vi "PeakAll.vi"(11 "POTTypedCircularBuffer in":refnum<class "ErrorLogBuffer.lvclass">) -> (2 "Copied Buffer":T1[](array[typedef]), 3 "POTTypedCircularBuffer out":refnum<class "ErrorLogBuffer.lvclass">)   [LabVIEW 2024, in "ErrorLogBuffer.lvclass"]
uses:
  ErrorLogBuffer.lvclass
  Type.ctl
  RQMHCore/ErrorReporting/Record/LogRecord.lvclass
  ErrorLogBuffer.lvclass/ErrorLogBuffer.ctl
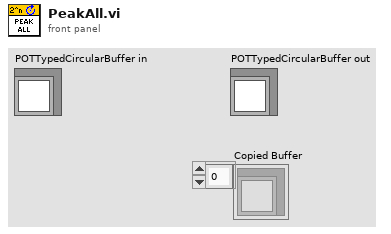
[diagram p1: front panel]
types:
  T1 = typedef "ErrorLogBuffer.lvclass/Type.ctl" = refnum<class "LogRecord.lvclass">
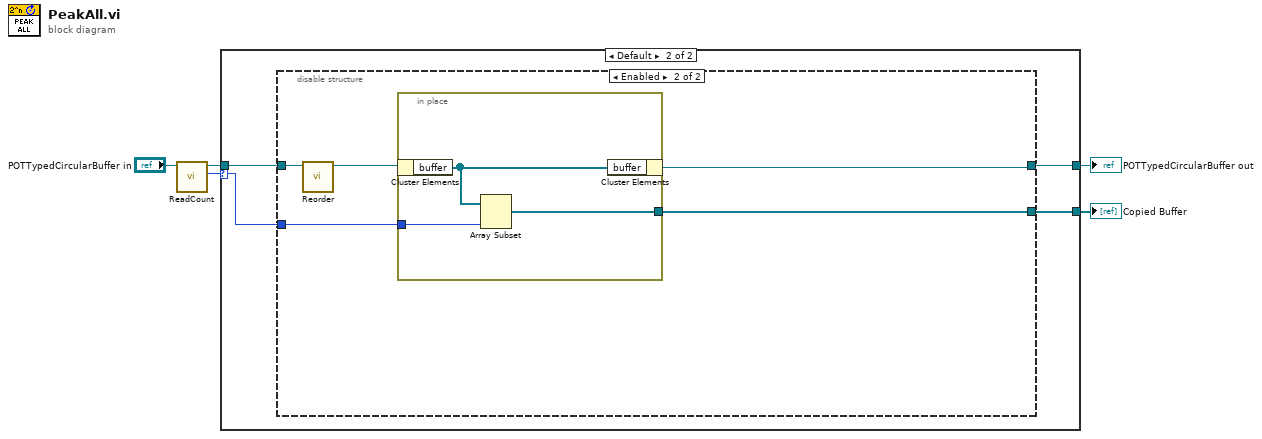
[diagram p0: block diagram]
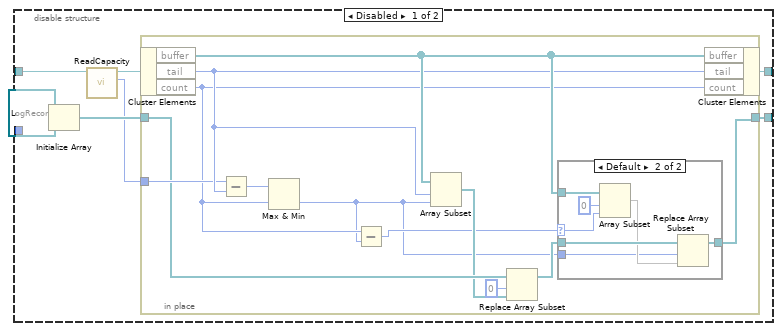
[diagram p3: hidden frame]
diagram:
  n1 = call "ReadCount.vi"("POTTypedCircularBuffer in"="POTTypedCircularBuffer in") -> ("count"=w1:i32, "POTTypedCircularBuffer out"=w2:refnum<class "ErrorLogBuffer.lvclass">)  [unwired: 9 in]
  n2 = case shown="Default" w1 {
    selector: w1 -> [_ w7]
    tunnel: [w6 w10] -> w5
    tunnel: [_ w9] -> w4
    tunnel: w2 -> [w6 w8]
    frame 0 {
    }
    frame Default {
      n3 = disable-structure shown="Enabled" {
        disable-tunnel: [w18 w39] -> w10
        disable-tunnel: [w17 w40] -> w9
        disable-tunnel: w8 -> [w14 w43]
        disable-tunnel: w7 -> [w11 w41]
        frame Disabled {
          n4 = Initialize Array(T1 refnum ("Type"), w11) -> (w15:T1[])
          n5 = call "ReadCapacity.vi"("POTTypedCircularBuffer in"=w14) -> ("capacity"=w12:i32, "POTTypedCircularBuffer out"=w13:refnum<class "ErrorLogBuffer.lvclass">)  [unwired: 9 in]
          n6 = in-place {
            in-place-border: [w26] -> w17
            in-place-border: w15 -> [w27]
            in-place-border: w12 -> [w28]
            n7 = in-place-cluster #1(w13) -> ("buffer"=w30:T1[], "tail"=w29:i32, "count"=w25:i32)
            n8 = Subtract(x=w28, y=w29) -> (x-y=w24:i32)
            n9 = Max & Min(x=w24, y=w25) -> (min(x,y)=w19:i32)  [unwired: 1 out]
            n10 = Subtract(x=w25, y=w19) -> (x-y=w20:i32)
            n11 = Array Subset(array=w30, index=w29, length=w19) -> (w22:T1[])
            n12 = Replace Array Subset(array=w27, new element=w22, index=0) -> (w21:T1[])
            n13 = case shown="Default" w20 {
              selector: w20 -> [_ w33]
              tunnel: w21 -> [w31 w38]
              tunnel: [w31 w37] -> w26
              tunnel: w30 -> [_ w36]
              tunnel: w19 -> [_ w32]
              frame 0 {
              }
              frame Default {
                n14 = Array Subset(array=w36, index=0, length=w33) -> (w34:T1[])
                n15 = Replace Array Subset(array=w38, new element=w34, index=w32) -> (w37:T1[])
              }
            }
            n16 = in-place-cluster #1("buffer"=w30, "tail"=w29, "count"=w25) -> (w18:refnum<class "ErrorLogBuffer.lvclass">)
          }
        }
        frame Enabled {
          n17 = call "Reorder.vi"("POTTypedCircularBuffer in"=w43) -> ("POTTypedCircularBuffer out"=w42:refnum<class "ErrorLogBuffer.lvclass">)  [unwired: 10 in]
          n18 = in-place {
            in-place-border: w41 -> [w46]
            in-place-border: [w45] -> w40
            n19 = in-place-cluster #2(w42) -> ("buffer"=w44:T1[])
            n20 = Array Subset(array=w44, length=w46) -> (w45:T1[])  [unwired: 1 in]
            n21 = in-place-cluster #2("buffer"=w44) -> (w39:refnum<class "ErrorLogBuffer.lvclass">)
          }
        }
      }
    }
  }
  "POTTypedCircularBuffer out" <- w5
  "Copied Buffer" <- w4
